vi "Do Fold.vi"(10 "Fold":T3, 11 "Puzzle In":T1) -> (3 "Puzzle":T1)   [LabVIEW 2020]
uses:
  Fold.ctl
  Axis.ctl
  Puzzle.ctl
  Dot.ctl
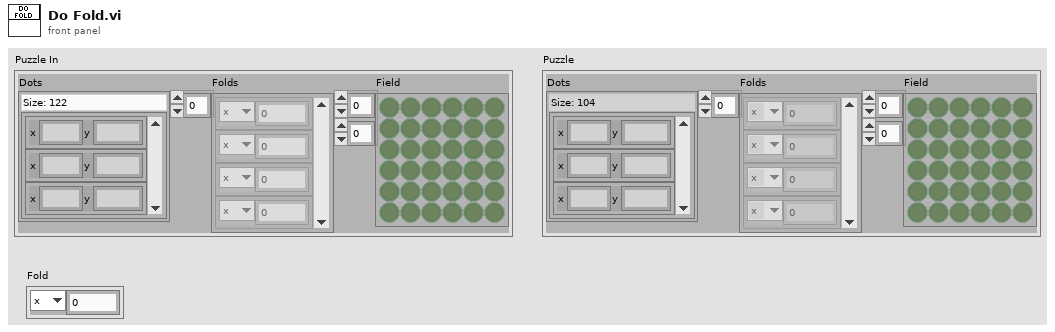
[diagram p1: front panel]
types:
  T1 = typedef "Puzzle.ctl" = cluster{"Dots":set{T2}, "Folds":T3[], "Field":bool[][]}
  T2 = typedef "Dot.ctl" = cluster{"x":i32, "y":i32}
  T3 = typedef "Fold.ctl" = cluster{"Axis":T4, "Value":i32}
  T4 = typedef "Axis.ctl" = enum16{"x", "y"}
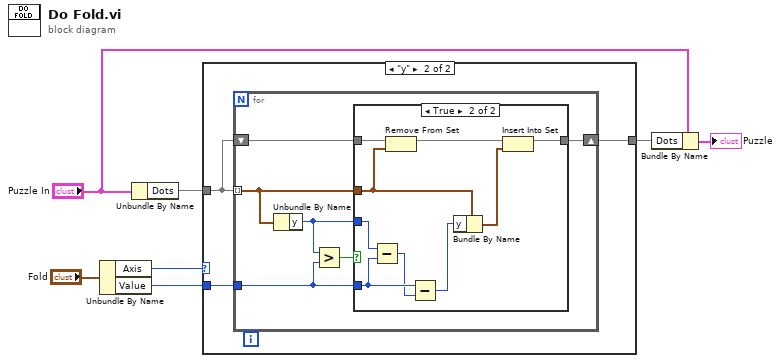
[diagram p0: block diagram]
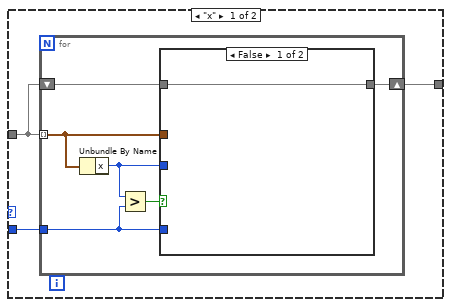
[diagram p2: hidden frame]
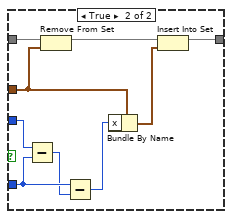
[diagram p3: hidden frame]
diagram:
  n1 = Unbundle By Name("Fold") -> ("Axis"=w6:T4, "Value"=w5:i32)
  n2 = Unbundle By Name("Puzzle In") -> ("Dots"=w4:set{T2})
  n3 = case shown="\"y\"" w6 {
    tunnel: w5 -> [w9 w28]
    tunnel: w4 -> [w10 w29]
    tunnel: [w8 w27] -> w1
    frame "x" {
      n4 = for {
        tunnel: w10 -> [w15] mode=indexing
        shift-right: [w11] -> w8
        shift-left: w10 -> [w14]
        tunnel: w9 -> [w12]
        n5 = Unbundle By Name(w15) -> ("x"=w13:i32)
        n6 = Greater?(x=w13, y=w12) -> (0:w16:bool)
        n7 = case shown="False" w16 {
          tunnel: w15 -> [_ w22]
          tunnel: w14 -> [w17 w26]
          tunnel: w13 -> [_ w25]
          tunnel: w12 -> [_ w24]
          tunnel: [w17 w18] -> w11
          frame False {
          }
          frame True {
            n8 = Subtract(x=w25, y=w24) -> (x-y=w23:i32)
            n9 = Remove From Set(10:w22, 11:w26) -> (3:w20:set{T2})  [unwired: 1 out]
            n10 = Subtract(x=w24, y=w23) -> (x-y=w21:i32)
            n11 = Bundle By Name(cluster=w22, "x"=w21) -> (w19:T2)
            n12 = Insert Into Set(10:w19, 11:w20) -> (3:w18:set{T2})  [unwired: 1 out]
          }
        }
      }
    }
    frame "y" {
      n13 = for {
        tunnel: w29 -> [w34] mode=indexing
        shift-right: [w30] -> w27
        shift-left: w29 -> [w33]
        tunnel: w28 -> [w31]
        n14 = Unbundle By Name(w34) -> ("y"=w32:i32)
        n15 = Greater?(x=w32, y=w31) -> (0:w35:bool)
        n16 = case shown="True" w35 {
          tunnel: w34 -> [_ w41]
          tunnel: w33 -> [w36 w45]
          tunnel: w32 -> [_ w44]
          tunnel: w31 -> [_ w43]
          tunnel: [w36 w37] -> w30
          frame False {
          }
          frame True {
            n17 = Subtract(x=w44, y=w43) -> (x-y=w42:i32)
            n18 = Remove From Set(10:w41, 11:w45) -> (3:w39:set{T2})  [unwired: 1 out]
            n19 = Subtract(x=w43, y=w42) -> (x-y=w40:i32)
            n20 = Bundle By Name(cluster=w41, "y"=w40) -> (w38:T2)
            n21 = Insert Into Set(10:w38, 11:w39) -> (3:w37:set{T2})  [unwired: 1 out]
          }
        }
      }
    }
  }
  n22 = Bundle By Name(cluster="Puzzle In", "Dots"=w1) -> (→"Puzzle":T1)
